vi "my rio motor.vi"() -> ()   [LabVIEW 2015]
uses:
  <vilib>/myRIO/Common/Instrument Driver Framework/myRIO v1.0/Encoder/typedefs/Encoder Count Direction Enum.ctl
  <vilib>/myRIO/Instrument Drivers/Onboard IO/Encoder/vis/Read.vi
  <vilib>/myRIO/Instrument Drivers/Onboard IO/PWM/vis/Set Duty Cycle and Frequency.vi
  <vilib>/myRIO/Instrument Drivers/Onboard IO/DIO/vis/Write.vi
  <vilib>/myRIO/Common/Instrument Driver Framework/myRIO v1.0/UART/vis/myRIO v1.0 Close UART.vi
  <vilib>/myRIO/Instrument Drivers/Onboard IO/Encoder/vis/Smart Open.vi
  <vilib>/Utility/error.llb/Error Cluster From Error Code.vi
  <vilib>/myRIO/Common/Instrument Driver Framework/myRIO v1.0/Encoder/vis/myRIO v1.0 Read Encoder.vi
  <vilib>/myRIO/Instrument Drivers/Onboard IO/PWM/vis/Smart Open.vi
  <vilib>/myRIO/Common/Instrument Driver Framework/myRIO v1.0/PWM/vis/myRIO v1.0 Write PWM.vi
  <vilib>/myRIO/Instrument Drivers/Onboard IO/DIO/vis/Smart Open.vi
  <vilib>/myRIO/Common/Instrument Driver Framework/myRIO v1.0/DIO/vis/myRIO v1.0 Write DIO.vi
  <vilib>/myRIO/Common/Instrument Driver Framework/Utilities/vis/FPGA Ref Manager.vi
  <vilib>/myRIO/Common/Instrument Driver Framework/myRIO v1.0/myRIO v1.0 Reset FPGA.vi
  <vilib>/myRIO/Common/Instrument Driver Framework/myRIO v1.0/IRQ/vis/myRIO v1.0 IRQ Info FGV.vi
  <vilib>/myRIO/Common/Instrument Driver Framework/myRIO v1.0/IRQ/vis/myRIO v1.0 Timer IRQ Info FGV.vi
  <vilib>/myRIO/Common/Instrument Driver Framework/myRIO v1.0/IRQ/vis/myRIO v1.0 ISR Agent.vi
  <vilib>/myRIO/Instrument Drivers/Utilities/Utilities.lvlib
panel:
  in  "[ESC]":bool
  in  "PWM freq [Hz]":dbl(slide)=100.0 scale=10.0..1000.0
  in  "PWM duty  [%]":dbl(slide) scale=-100.0..100.0
  in  "Enable":bool
  out "Direction":bool
  out "Counter Value":i32
  out "Counter Direction":T1
  in  "Reset Counter":bool
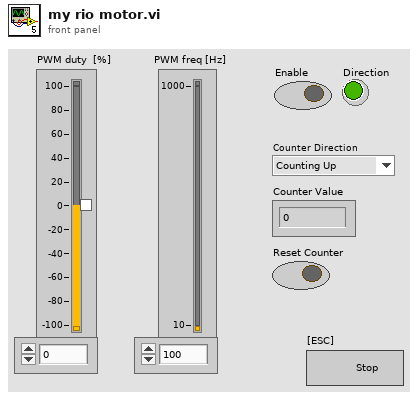
[diagram p1: front panel]
types:
  T1 = typedef "Encoder Count Direction Enum.ctl" = enum16{"Counting Up", "Counting Down"}
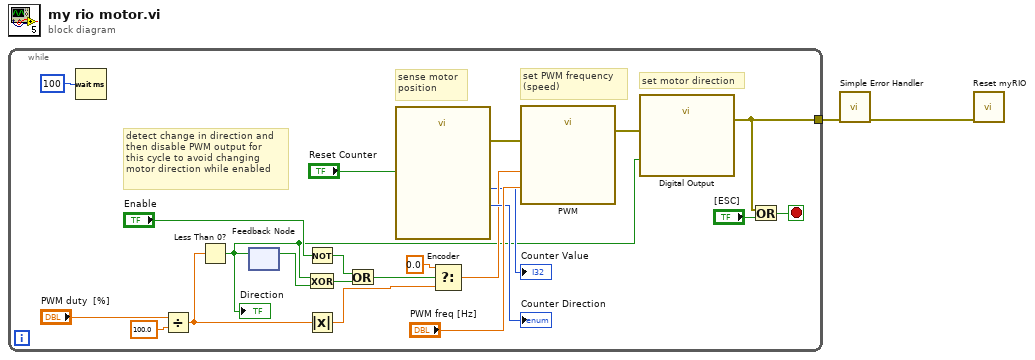
[diagram p0: block diagram]
diagram:
  n1 = while {
    tunnel: [w16] -> w1
    stop <- w24 stop-if-true
    # "sense motor \nposition"
    # "detect change in direction and\nthen disable PWM output for\nthis cycle to avoid changing\nmotor direction while enabled"
    # "set PWM frequency\n(speed)"
    # "set motor direction"
    n2 = Wait (ms)(milliseconds to wait=u32 100) -> ()  [unwired: 1 out]
    n3 = Divide(x="PWM duty  [%]", y=100.0) -> (x/y=w8:dbl)
    n4 = Less Than 0?(x=w8) -> (x < 0?=w3:bool)
    "Direction" <- w3
    n5 = feedback-in #1(w3) -> ()
    n6 = feedback #1() -> (w18:bool)  [unwired: 1 in]
    n7 = Not(x="Enable") -> (.not. x?=w12:bool)
    n8 = Exclusive Or(1:w18, 2:w3) -> (0:w15:bool)
    n9 = Absolute Value(x=w8) -> (abs(x)=w5:dbl)
    n10 = Or(x=w12, y=w15) -> (x .or. y?=w14:bool)
    n11 = call "Encoder"("Reset Counter"="Reset Counter") -> ("Counter Value"=→"Counter Value":i32, "Counter Direction"=→"Counter Direction":T1, "error out"=w20:errorcluster)  [unwired: 23 in, 1 out]
    n12 = Select(t=0.0 ("f"), s=w14, f=w5) -> (s? t:f=w7:dbl)
    n13 = call "PWM"("Duty Cycle (0-1)"=w7, "Frequency (Hz)"="PWM freq [Hz]", "error in (no error)"=w20) -> ("error out"=w19:errorcluster)  [unwired: 24 in]
    n14 = call "Digital Output"("A/DIO0 (Pin 11)"=w3, "error in (no error)"=w19) -> ("error out"=w16:errorcluster)  [unwired: 25 in]
    n15 = Or(x=w16, y="[ESC]") -> (x .or. y?=w24:bool)
  }
  n16 = call <vilib>:"Simple Error Handler.vi"("error in (no error)"=w1) -> ("error out"=w2:errorcluster)  [unwired: 4 in, 4 out]
  n17 = call <vilib>:"Reset myRIO.vi"("error in (no error)"=w2) -> ()  [unwired: 10 in, 1 out]
